vi "AddSharedVariableToParent.vi"(6 "Variable Type (Network-Published)":T1(ring)=enum."Network-Published", 8 "error in (no error)":errorcluster, 9 "Variable Data Type (Double)":variant=variant(dbl 0.0), 10 "Variable Name":string, 11 "Library Reference In":refnum<vi>) -> (0 "error out":errorcluster, 2 "Variable Reference Out":refnum<vi>, 3 "Library Reference Out":refnum<vi>)   [LabVIEW 2017]
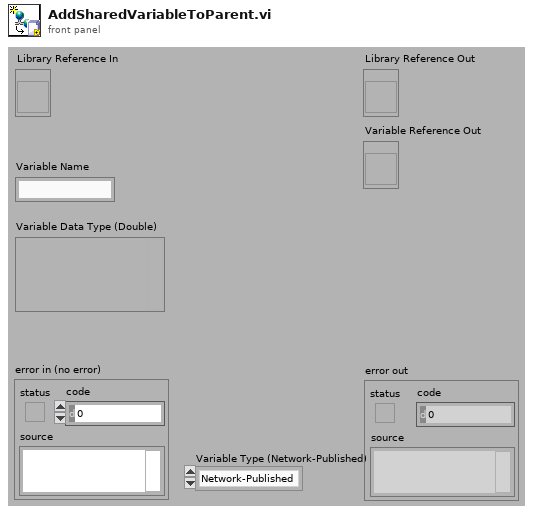
[diagram p1: front panel]
types:
  T1 = enum16{"Single-Process", "Network-Published", "Time-Triggered"}
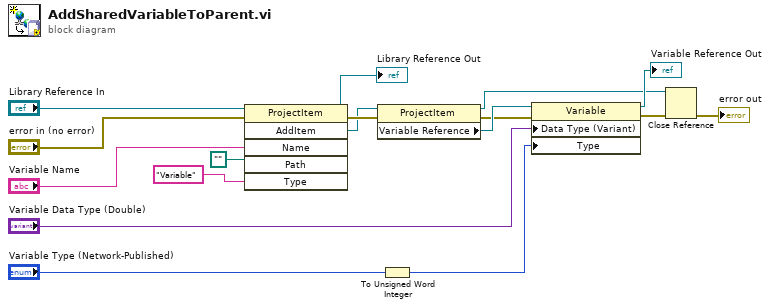
[diagram p0: block diagram]
diagram:
  n1 = invoke class="ProjectItem" method="AddItem"(reference="Library Reference In", error in="error in (no error)", "Name"="Variable Name", "Path"=path "", "Type"="Variable") -> (reference out=→"Library Reference Out":refnum<vi>, error out=w11:errorcluster, "AddItem"=w10:refnum<vi>)  [unwired: 1 in, 3 out]
  n2 = property class="ProjectItem"(reference=w10, error in=w11) -> (reference out=w3:refnum<vi>, error out=w8:errorcluster, "Variable Reference"=w9:refnum<vi>)
  n3 = To Unsigned Word Integer(number="Variable Type (Network-Published)") -> (unsigned 16bit integer=w1:u16)
  n4 = property class="Variable"(reference=w9, error in=w8, "Data Type (Variant)"="Variable Data Type (Double)", "Type"=w1) -> (reference out=→"Variable Reference Out":refnum<vi>, error out=w4:errorcluster)
  n5 = Close Reference(reference=w3, error in (no error)=w4) -> (error out=→"error out":errorcluster)
